vi "Launcher - Manager Panel.vi"(6 "Worker Alias":string="Manager Panel", 8 "error in":errorcluster, 9 "Initialization Data":T1, 11 "Manager Panel in":refnum<class "Manager Panel.lvclass">) -> (0 "error out":errorcluster)   [LabVIEW 2020]
doc: "This VI launches the Head Worker of a Workers application."
uses:
  Workers/Manager Panel/Initialization Data.ctl
  Workers/Manager Panel/Response Cases.ctl
  Workers/Manager Panel/Manager Panel.lvclass
  C:/Program Files (x86)/National Instruments/LabVIEW 2020/vi.lib/addons/_Workers/Library/Classes/Worker/Worker.lvclass
  <vilib>/addons/_Workers/Debugger/Debug Client/Debug Client.lvlib
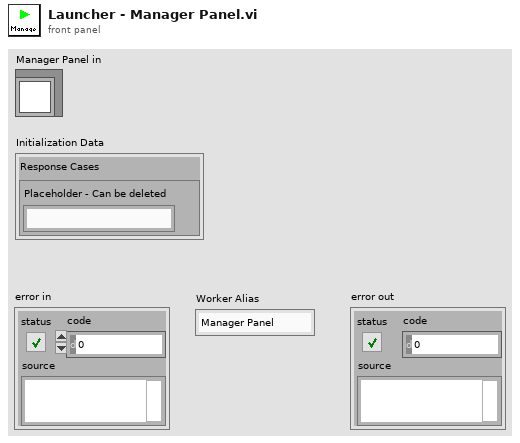
[diagram p1: front panel]
types:
  T1 = typedef "Manager Panel.lvclass/Initialization Data.ctl" = cluster{"Response Cases":T2}
  T2 = typedef "Manager Panel.lvclass/Response Cases.ctl" = cluster{"Placeholder - Can be deleted":string}
  T3 = enum32{"Invalid", "Standard", "Closed", "Hidden", "Minimized", "Maximized"}
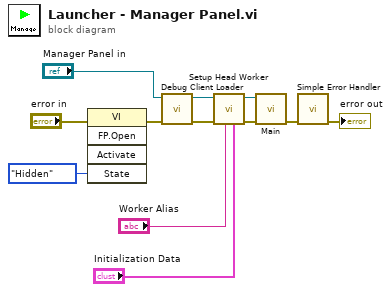
[diagram p0: block diagram]
diagram:
  n1 = invoke class="VI" method="FP.Open"(error in="error in", "State"=T3."Hidden" ("״̬")) -> (error out=w1:errorcluster)  [unwired: 3 in, 4 out]
  n2 = call <vilib>:"Debug Client Loader.vi"("error in (no error)"=w1, "Worker_"="Manager Panel in") -> ("error out"=w6:errorcluster, "Worker_out"=w4:refnum<class "Manager Panel.lvclass">)  [unwired: 8 in]
  n3 = call-dynamic "Setup Head Worker.vi"("Initalization Data"="Initialization Data", "Worker Alias"="Worker Alias", "error in"=w6, "Worker_"=w4) -> ("error out"=w12:errorcluster, "Worker_out"=w10:refnum<class "Manager Panel.lvclass">)  [unwired: 6 in]
  n4 = call-dynamic "Main.vi"("error in"=w12, "Manager Panel in"=w10) -> ("error out"=w11:errorcluster)  [unwired: 8 in, 1 out]
  n5 = call <vilib>:"Simple Error Handler.vi"("error in (no error)"=w11) -> ("error out"=→"error out":errorcluster)  [unwired: 4 in, 4 out]
